vi "BuildWorker Tester.vi"() -> ()   [LabVIEW 2017]
uses:
  src/LabVIEW/vi.lib/BenjaminR/Build Farm/Classes/Task Interface/Task/Task.lvclass
  src/LabVIEW/vi.lib/BenjaminR/Build Farm/Actors/Communication/Connection Listener/Connection Listener/Connection Listener.lvclass/Connection Listener.ctl
  src/LabVIEW/vi.lib/BenjaminR/Build Farm/Actors/Communication/Connection Listener/Connection Listener Messages/Forward Message Msg/Forward Message Msg.lvclass/Forward Message Msg.ctl
  <vilib>/ActorFramework/Message Enqueuer/Message Enqueuer.lvclass/Message Enqueuer.ctl
  src/LabVIEW/vi.lib/BenjaminR/Build Farm/Actors/Communication/Connection Listener/Connection Listener/Read Msg Update.vi
  <vilib>/ActorFramework/Message Enqueuer/Enqueue.vi
  src/LabVIEW/vi.lib/BenjaminR/Build Farm/Actors/Communication/Connection Listener/Connection Listener/Connection Listener.lvclass
  C:/Program Files (x86)/National Instruments/LabVIEW 2017/vi.lib/ActorFramework/Actor/Actor.lvclass
  src/LabVIEW/vi.lib/BenjaminR/Build Farm/Actors/Communication/Connection Listener/Connection Listener Messages/Forward Message Msg/Forward Message Msg.lvclass
  C:/Program Files (x86)/National Instruments/LabVIEW 2017/vi.lib/ActorFramework/Message/Message.lvclass
  <vilib>/ActorFramework/Stop Msg/Stop Msg.lvclass
  <vilib>/ActorFramework/Message Priority Queue/Priority Enqueue.vi
  <vilib>/ActorFramework/Actor/Actor.lvclass
  src/LabVIEW/vi.lib/BenjaminR/Build Farm/Actors/Communication/Connection Listener/Connection Listener Messages/Get Connection List Msg/Get Connection List Msg.lvclass
  src/LabVIEW/vi.lib/BenjaminR/Build Farm/Classes/Message Interface/Command/Command.lvclass
panel:
  out "status":string
  in  "abort":bool
  in  "start":bool
  out "Task out":refnum<class "Task.lvclass">
  in  "removeTask":bool
  in  "Name":string
  in  "ProjectPath":path
  in  "BuildSpec Name":string
  in  "Target":string
  in  "newTask":bool
  in  "name":bool
  in  "taskName":bool
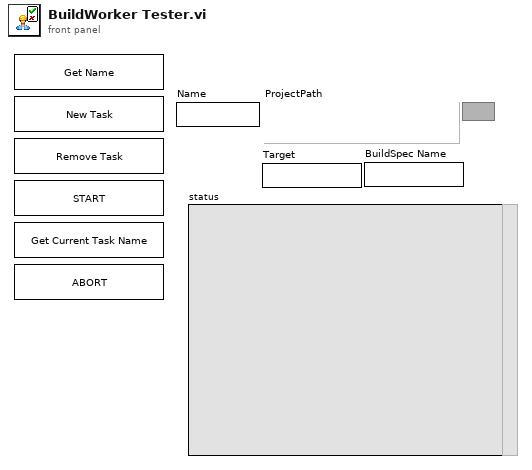
[diagram p1: front panel]
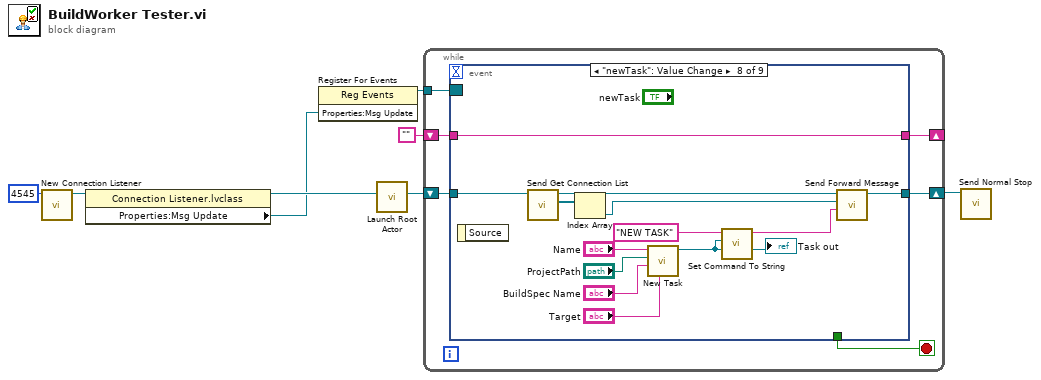
[diagram p0: block diagram]
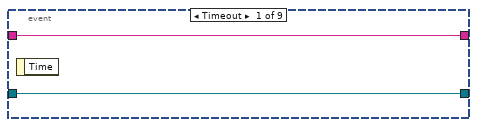
[diagram p2: hidden frame]
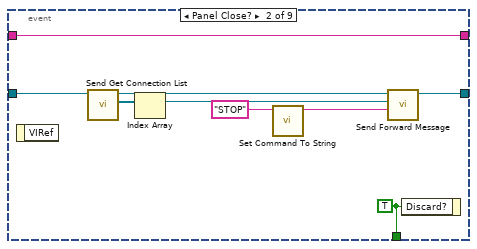
[diagram p3: hidden frame]
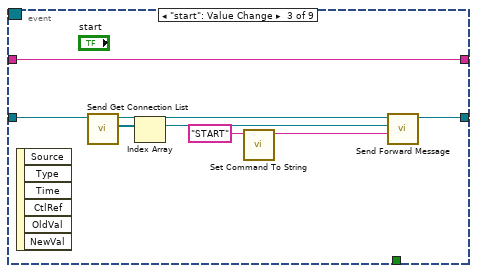
[diagram p4: hidden frame]
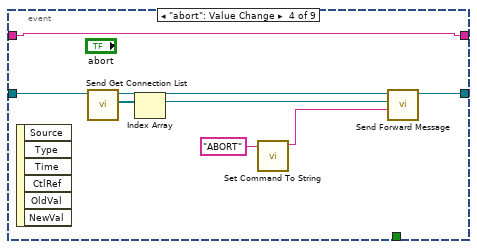
[diagram p5: hidden frame]
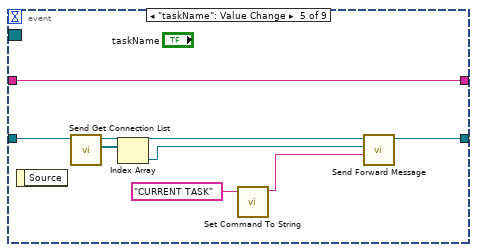
[diagram p6: hidden frame]
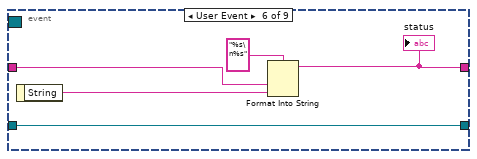
[diagram p7: hidden frame]
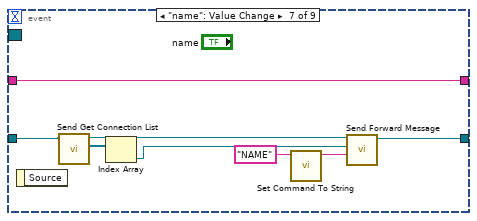
[diagram p8: hidden frame]
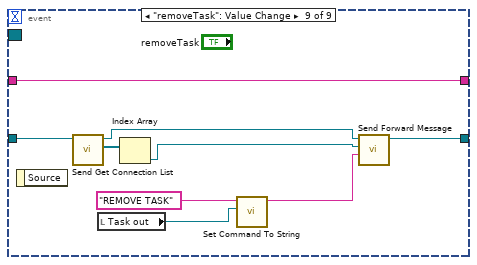
[diagram p9: hidden frame]
diagram:
  n1 = call "New Connection Listener.vi"("Port"=u16 4545 ("BuildServer Name")) -> ("Connection Listener out"=w1:refnum<class "Connection Listener.lvclass">)  [unwired: 9 in, 1 out]
  n2 = property class="Connection Listener.lvclass"(reference=w1) -> (reference out=w6:refnum<class "Connection Listener.lvclass">, "Properties:Msg Update"=w4:refnum<user-event>)  [unwired: 1 in, 1 out]
  n3 = register-events(w4) -> (reference out=w5:refnum<event-registration>)  [unwired: 2 in, 1 out]
  n4 = call <vilib>:"Launch Root Actor.vi"("Actor"=w6) -> ("Actor's Enqueuer"=w7:refnum<class "Message Enqueuer.lvclass">)  [unwired: 9 in, 1 out]
  n5 = while {
    shift-right: [w12] -> w8
    shift-left: w7 -> [w13]
    tunnel: w5 -> [w11]
    shift-right: [w9] -> _
    shift-left: "" -> [w10]
    stop <- w14 stop-if-true
    n6 = event shown="[7] \"newTask\": Value Change" {
      selector: w11 -> [_ _ _ _ _ _ _ _ _]
      dyn-events: _ -> [_ _ _ _ _ _ _ _ _]
      timeout: _ -> [_ _ _ _ _ _ _ _ _]
      tunnel: [_ w25 _ _ _ _ _ _ _] -> w14
      tunnel: w13 -> [w16 w23 w32 w40 w47 w54 w60 w69 w82]
      tunnel: [w16 w24 w33 w41 w49 w54 w62 w71 w84] -> w12
      tunnel: w10 -> [w15 w19 w28 w36 w44 w52 w57 w66 w79]
      tunnel: [w15 w19 w28 w36 w44 w51 w57 w66 w79] -> w9
      event Timeout {
        n7 = event-data() -> ()  [unwired: 1 in, 1 out]
      }
      event Panel Close? {
        w25 = TRUE ("Discard?")
        n8 = event-data() -> ()  [unwired: 1 in, 1 out]
        n9 = call "Send Get Connection List.vi"("Message Enqueuer in"=w23) -> ("Connection List"=w21:refnum<class "Message Enqueuer.lvclass">[], "Message Enqueuer out"=w22:refnum<class "Message Enqueuer.lvclass">)  [unwired: 8 in, 1 out]
        n10 = Index Array(array=w21) -> (element=w20:refnum<class "Message Enqueuer.lvclass">)  [unwired: 1 in]
        n11 = call "Set Command To String.vi"("Command"="STOP") -> ("data string"=w17:string)  [unwired: 10 in]
        n12 = call "Send Forward Message.vi"("Message"=w17, "Dest Enqueuer"=w20, "Message Enqueuer in"=w22) -> ("Message Enqueuer out"=w24:refnum<class "Message Enqueuer.lvclass">)  [unwired: 7 in, 1 out]
        n13 = event-data("Discard?"=w25) -> ()  [unwired: 1 in, 1 out]
      }
      event "start": Value Change {
        n14 = event-data() -> ()  [unwired: 1 in, 6 out]
        n15 = call "Send Get Connection List.vi"("Message Enqueuer in"=w32) -> ("Connection List"=w30:refnum<class "Message Enqueuer.lvclass">[], "Message Enqueuer out"=w31:refnum<class "Message Enqueuer.lvclass">)  [unwired: 8 in, 1 out]
        n16 = Index Array(array=w30) -> (element=w29:refnum<class "Message Enqueuer.lvclass">)  [unwired: 1 in]
        n17 = call "Set Command To String.vi"("Command"="START") -> ("data string"=w26:string)  [unwired: 10 in]
        n18 = call "Send Forward Message.vi"("Message"=w26, "Dest Enqueuer"=w29, "Message Enqueuer in"=w31) -> ("Message Enqueuer out"=w33:refnum<class "Message Enqueuer.lvclass">)  [unwired: 7 in, 1 out]
      }
      event "abort": Value Change {
        n19 = event-data() -> ()  [unwired: 1 in, 6 out]
        n20 = call "Send Get Connection List.vi"("Message Enqueuer in"=w40) -> ("Connection List"=w38:refnum<class "Message Enqueuer.lvclass">[], "Message Enqueuer out"=w39:refnum<class "Message Enqueuer.lvclass">)  [unwired: 8 in, 1 out]
        n21 = Index Array(array=w38) -> (element=w37:refnum<class "Message Enqueuer.lvclass">)  [unwired: 1 in]
        n22 = call "Set Command To String.vi"("Command"="ABORT") -> ("data string"=w34:string)  [unwired: 10 in]
        n23 = call "Send Forward Message.vi"("Message"=w34, "Dest Enqueuer"=w37, "Message Enqueuer in"=w39) -> ("Message Enqueuer out"=w41:refnum<class "Message Enqueuer.lvclass">)  [unwired: 7 in, 1 out]
      }
      event "taskName": Value Change {
        n24 = event-data() -> ()  [unwired: 1 in, 1 out]
        n25 = call "Send Get Connection List.vi"("Message Enqueuer in"=w47) -> ("Connection List"=w48:refnum<class "Message Enqueuer.lvclass">[], "Message Enqueuer out"=w46:refnum<class "Message Enqueuer.lvclass">)  [unwired: 8 in, 1 out]
        n26 = Index Array(array=w48) -> (element=w45:refnum<class "Message Enqueuer.lvclass">)  [unwired: 1 in]
        n27 = call "Set Command To String.vi"("Command"="CURRENT TASK") -> ("data string"=w42:string)  [unwired: 10 in]
        n28 = call "Send Forward Message.vi"("Message"=w42, "Dest Enqueuer"=w45, "Message Enqueuer in"=w46) -> ("Message Enqueuer out"=w49:refnum<class "Message Enqueuer.lvclass">)  [unwired: 7 in, 1 out]
      }
      event User Event {
        n29 = event-data() -> ("String"=w50:string)  [unwired: 1 in]
        n30 = Format Into String(format string="%s\n%s", w52, w50) -> (resulting string=w51:string)  [unwired: 2 in, 1 out]
        "status" <- w51
      }
      event "name": Value Change {
        n31 = event-data() -> ()  [unwired: 1 in, 1 out]
        n32 = call "Send Get Connection List.vi"("Message Enqueuer in"=w60) -> ("Connection List"=w61:refnum<class "Message Enqueuer.lvclass">[], "Message Enqueuer out"=w59:refnum<class "Message Enqueuer.lvclass">)  [unwired: 8 in, 1 out]
        n33 = Index Array(array=w61) -> (element=w58:refnum<class "Message Enqueuer.lvclass">)  [unwired: 1 in]
        n34 = call "Set Command To String.vi"("Command"="NAME") -> ("data string"=w55:string)  [unwired: 10 in]
        n35 = call "Send Forward Message.vi"("Message"=w55, "Dest Enqueuer"=w58, "Message Enqueuer in"=w59) -> ("Message Enqueuer out"=w62:refnum<class "Message Enqueuer.lvclass">)  [unwired: 7 in, 1 out]
      }
      event "newTask": Value Change {
        n36 = event-data() -> ()  [unwired: 1 in, 1 out]
        n37 = call "Send Get Connection List.vi"("Message Enqueuer in"=w69) -> ("Connection List"=w70:refnum<class "Message Enqueuer.lvclass">[], "Message Enqueuer out"=w68:refnum<class "Message Enqueuer.lvclass">)  [unwired: 8 in, 1 out]
        n38 = Index Array(array=w70) -> (element=w67:refnum<class "Message Enqueuer.lvclass">)  [unwired: 1 in]
        n39 = call "New Task.vi"("Target"="Target", "BuildSpec Name"="BuildSpec Name", "ProjectPath"="ProjectPath", "Name"="Name") -> ("Task out"=w64:refnum<class "Task.lvclass">)  [unwired: 6 in, 1 out]
        "Task out" <- w64
        n40 = call "Set Command To String.vi"("Arguments"=w64, "Command"="NEW TASK") -> ("data string"=w63:string)  [unwired: 9 in]
        n41 = call "Send Forward Message.vi"("Message"=w63, "Dest Enqueuer"=w67, "Message Enqueuer in"=w68) -> ("Message Enqueuer out"=w71:refnum<class "Message Enqueuer.lvclass">)  [unwired: 7 in, 1 out]
      }
      event "removeTask": Value Change {
        n42 = event-data() -> ()  [unwired: 1 in, 1 out]
        n43 = call "Send Get Connection List.vi"("Message Enqueuer in"=w82) -> ("Connection List"=w83:refnum<class "Message Enqueuer.lvclass">[], "Message Enqueuer out"=w81:refnum<class "Message Enqueuer.lvclass">)  [unwired: 8 in, 1 out]
        n44 = local read "Task out"() -> (w77:refnum<class "Task.lvclass">)
        n45 = Index Array(array=w83) -> (element=w80:refnum<class "Message Enqueuer.lvclass">)  [unwired: 1 in]
        n46 = call "Set Command To String.vi"("Arguments"=w77, "Command"="REMOVE TASK") -> ("data string"=w76:string)  [unwired: 9 in]
        n47 = call "Send Forward Message.vi"("Message"=w76, "Dest Enqueuer"=w80, "Message Enqueuer in"=w81) -> ("Message Enqueuer out"=w84:refnum<class "Message Enqueuer.lvclass">)  [unwired: 7 in, 1 out]
      }
    }
  }
  n48 = call <vilib>:"Send Normal Stop.vi"("Message Enqueuer"=w8) -> ()  [unwired: 10 in, 1 out]
